vi "DEPRACATED Get Nested Object Item by Name Array.vi"(7 "Item Path (as array of names)":string[](array[string]), 8 "error in (no error)":errorcluster, 10 "Object Offset":i32, 11 "JSON":string) -> (0 "error out":errorcluster, 1 "Offset past Item (or past last Item, if not found)":i32, 2 "Item Offset (-1 if not found)":i32, 3 "Found":bool)   [LabVIEW 2013, in "JSONtext.lvlib"]
uses:
  JSONtext.lvlib
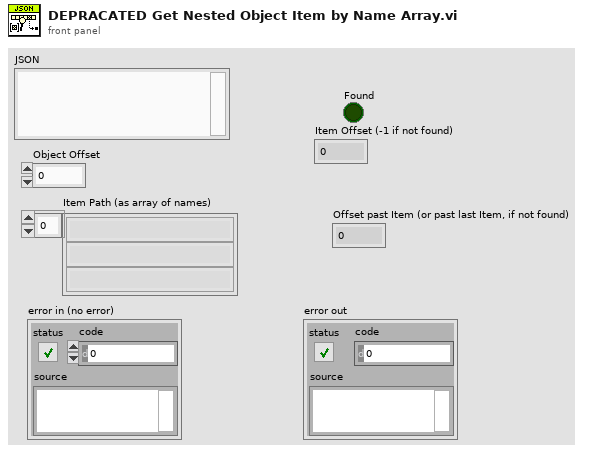
[diagram p1: front panel]
types:
  T1 = typedef "JSONtext.lvlib/Parsing State.ctl" = enum16{"Parser Error", "Object", "Array", "String", "Number/Other", "Leading Whitespace", "Object end", "Array end", "Value end"}
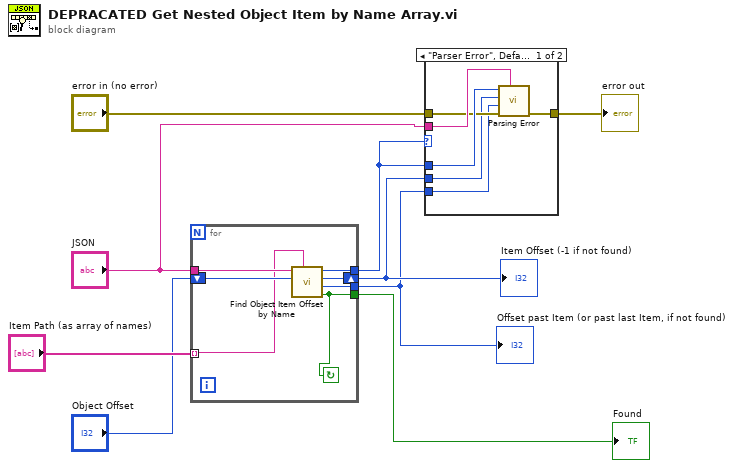
[diagram p0: block diagram]
diagram:
  n1 = for {
    tunnel: [w11] -> w9
    tunnel: [w16] -> w8
    tunnel: "JSON" -> [w15]
    tunnel: [w13] -> w3
    tunnel: "Item Path (as array of names)" -> [w10] mode=indexing
    shift-right: [w14] -> w4
    shift-left: "Object Offset" -> [w12]
    stop <- w11 continue-if-true
    n2 = call "Find Object Item Offset by Name.vi"("Item Name <JSON>"=w10, "Object Offset"=w12, "JSON"=w15) -> ("Found"=w11:bool, "Offset past Item (or past last Item, if not found)"=w13:i32, "Item Offset (-1 if not found)"=w14:i32, "State"=w16:T1)  [unwired: 4 in, 1 out]
  }
  "Found" <- w9
  "Item Offset (-1 if not found)" <- w4
  "Offset past Item (or past last Item, if not found)" <- w3
  n3 = case shown="\"Parser Error\", Default" w8 {
    tunnel: w8 -> [w22 _]
    tunnel: "JSON" -> [w21 _]
    tunnel: "error in (no error)" -> [w20 w23]
    tunnel: [w19 w23] -> w6
    tunnel: w4 -> [w18 _]
    tunnel: w3 -> [w17 _]
    frame "Parser Error", Default {
      n4 = call "Parsing Error.vi"("JSON"=w21, "error in (no error)"=w20, "Offset past match"=w17, "Value start"=w18, "State"=w22) -> ("error out"=w19:errorcluster)  [unwired: 6 in]
    }
    frame "Value end" {
    }
  }
  "error out" <- w6
